vi "HandleExit.vi"(8 "error in (no error)":errorcluster, 9 "VI Refnum":refnum<vi>, 10 "StopArgument":variant, 11 "ModuleAdmin":refnum<class "ModuleAdmin.lvclass">) -> (0 "error out":errorcluster, 1 "Exit via Stop Module Req?":bool, 2 "WaitForStop?":bool)   [LabVIEW 2017, in "NetworkImpairmentModule.lvlib"]
uses:
  NetworkImpairmentModule.lvlib
  <userlib>/NIST/ModuleAdminLib/ModuleAdmin/ModuleAdmin.lvclass
  C:/Program Files (x86)/National Instruments/LabVIEW 2017/user.lib/NIST/ModuleAdminLib/ModuleAdminBase/ModuleAdminBase.lvclass
  PublicAPI/Arguments/Requests/clStopArgument.ctl
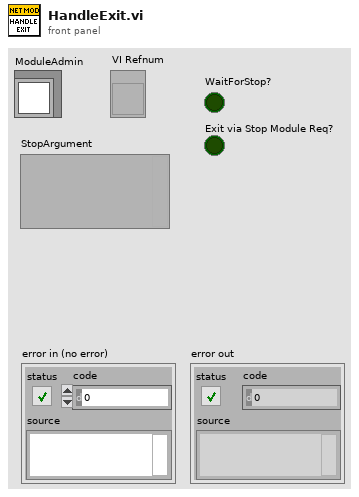
[diagram p1: front panel]
types:
  T1 = typedef "NetworkImpairmentModule.lvlib/clStopArgument.ctl" = cluster{"Exit via Stop Module Req?":bool, "Wait for Module to stop?":bool, "ModuleAdmin":refnum<class "ModuleAdmin.lvclass">}
  T2 = enum32{"Invalid", "Standard", "Closed", "Hidden", "Minimized", "Maximized"}
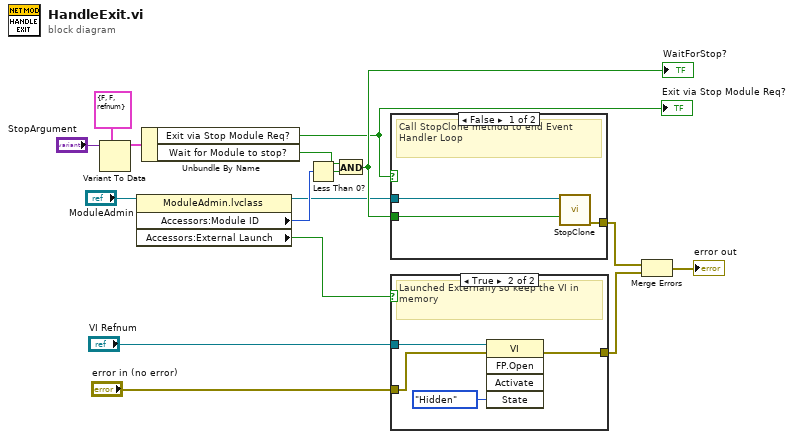
[diagram p0: block diagram]
diagram:
  n1 = Variant To Data(type=T1 {"Exit via Stop Module Req?"=FALSE, "Wait for Module to stop?"=FALSE, "ModuleAdmin"=refnum} ("Stop Argument"), Variant="StopArgument") -> (data=w8:T1)  [unwired: 1 in, 1 out]
  n2 = property class="ModuleAdmin.lvclass"(reference="ModuleAdmin") -> (reference out=w2:refnum<class "ModuleAdmin.lvclass">, "Accessors:Module ID"=w5:i32, "Accessors:External Launch"=w1:bool)  [unwired: 1 in, 1 out]
  n3 = Unbundle By Name(w8) -> ("Exit via Stop Module Req?"=w3:bool, "Wait for Module to stop?"=w4:bool)
  "Exit via Stop Module Req?" <- w3
  n4 = Less Than 0?(x=w5) -> (x < 0?=w15:bool)
  n5 = And(x=w4, y=w15) -> (x .and. y?=w6:bool)
  "WaitForStop?" <- w6
  n6 = case shown="False" w3 {
    tunnel: [w19 _] -> w12
    tunnel: w6 -> [w18 _]
    tunnel: w2 -> [w17 _]
    frame False {
      # "Call StopClone method to end Event Handler Loop"
      n7 = call "StopClone.vi"("Wait for Module to stop?"=w18, "ModuleAdmin"=w17) -> ("error out"=w19:errorcluster)  [unwired: 9 in]
    }
    frame True {
      # "This came from the Event Handler Loop"
    }
  }
  n8 = case shown="True" w1 {
    tunnel: "VI Refnum" -> [_ w24]
    tunnel: [w20 w22] -> w11
    tunnel: "error in (no error)" -> [w20 w21]
    frame False {
    }
    frame True {
      # "Launched Externally so keep the VI in memory"
      n9 = invoke class="VI" method="FP.Open"(reference=w24, error in=w21, "State"=T2."Hidden") -> (error out=w22:errorcluster)  [unwired: 2 in, 4 out]
    }
  }
  n10 = Merge Errors(w12, w11) -> (→"error out":errorcluster)
